vi "Import Export - Unflatten from XML (CAR fix).vi"(8 "Error In":errorcluster, 10 "XML String In":string) -> (0 "Error Out":errorcluster, 2 "Import":T1 {"Tree"."Properties"."Type" items=["K_STRING", "K_BOOL", "K_I32", "K_U32", "K_DOUBLE", "K_U64", "K_VARIANT", "K_DEPENDENTFILE", "K_DEPENDENTNODE", "K_DATASOURCENODE", "K_U16", "K_DBLARR", "K_U32ARR", "K_I32ARR", "K_STRINGARR", "K_DICTIONARY", "K_DICTIONARYARR"]})   [LabVIEW 2017, in "PXImc System Explorer.lvlib"]
doc: "Unflattern XML to Import data. It contains a workaround the CAR #198717."
uses:
  PXImc System Explorer.lvlib
  <vilib>/NI/NI VeriStand Advanced SysDef API/_Types/SysDef.Export.ctl
  <vilib>/NI/NI VeriStand Advanced SysDef API/_Types/TreeItem.ctl
  <vilib>/NI/NI VeriStand Advanced SysDef API/_Types/TreeItem.Info.ctl
  <vilib>/NI Veristand/Custom Device API/Custom Device Channel.ctl
  <vilib>/NI Veristand/Custom Device API/Custom Device Channel Type.ctl
  <vilib>/NI Veristand/Custom Device API/Custom Device Waveform.ctl
  <vilib>/NI Veristand/Custom Device API/Custom Device Waveform DataType.ctl
  <vilib>/NI/NI VeriStand Advanced SysDef API/_Types/TreeItem.Property.ctl
  <vilib>/NI VeriStand/Custom Device API/Custom Device API.lvlib
  <vilib>/NI/NI VeriStand Advanced SysDef API/SysDef API/Advanced System Definition.lvlib
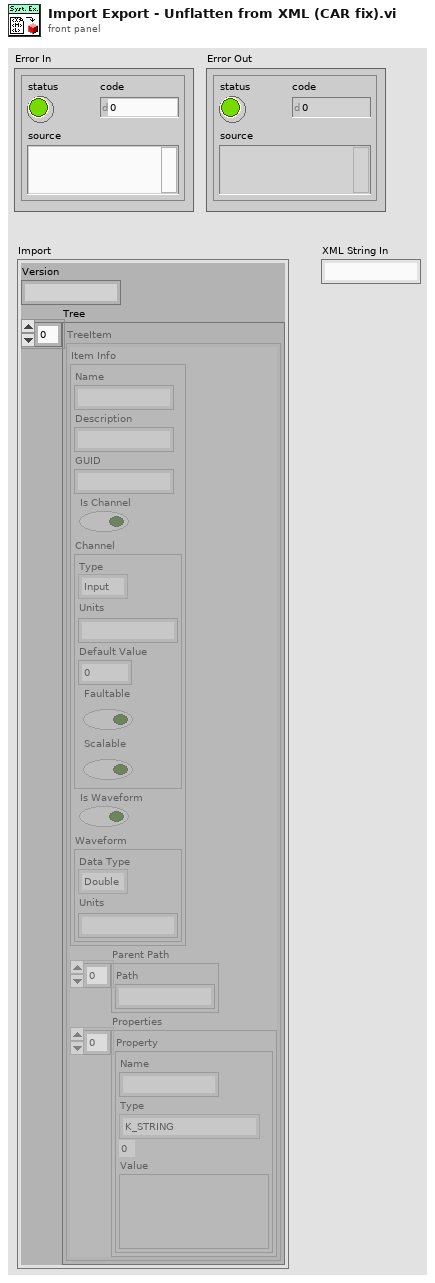
[diagram p1: front panel]
types:
  T1 = typedef "Advanced System Definition.lvlib/SysDef.Export.ctl" = cluster{"Version":string, "Tree":T2[]}
  T2 = typedef "Advanced System Definition.lvlib/TreeItem.ctl" = cluster{"Item Info":T3, "Parent Path":string[], "Properties":T8[]}
  T3 = typedef "Advanced System Definition.lvlib/TreeItem.Info.ctl" = cluster{"Name":string, "Description":string, "GUID":string, "Is Channel":bool, "Channel":T4, "Is Waveform":bool, "Waveform":T6}
  T4 = typedef "Custom Device API.lvlib/Custom Device Channel.ctl" = cluster{"Type":T5, "Units":string, "Default Value":dbl, "Faultable":bool, "Scalable":bool}
  T5 = typedef "Custom Device API.lvlib/Custom Device Channel Type.ctl" = enum16{"Input", "Output"}
  T6 = typedef "Custom Device API.lvlib/Custom Device Waveform.ctl" = cluster{"Data Type":T7, "Units":string}
  T7 = typedef "Custom Device API.lvlib/Custom Device Waveform DataType.ctl" = enum16{"Double", "Complex Double"}
  T8 = typedef "Advanced System Definition.lvlib/TreeItem.Property.ctl" = cluster{"Name":string, "Type":i32, "Value":variant}
  T9 = cluster{"Version":string, cluster{"Item Info":T3, "Parent Path":string[], cluster{"Name":string, "Type":i32, cluster{"type string":i16[], "data string":string}}[]}[]}
  T10 = cluster{"Item Info":T3, "Parent Path":string[], cluster{"Name":string, "Type":i32, cluster{"type string":i16[], "data string":string}}[]}[]
  T11 = cluster{"Name":string, "Type":i32, cluster{"type string":i16[], "data string":string}}[]
  T12 = cluster{"type string":i16[], "data string":string}
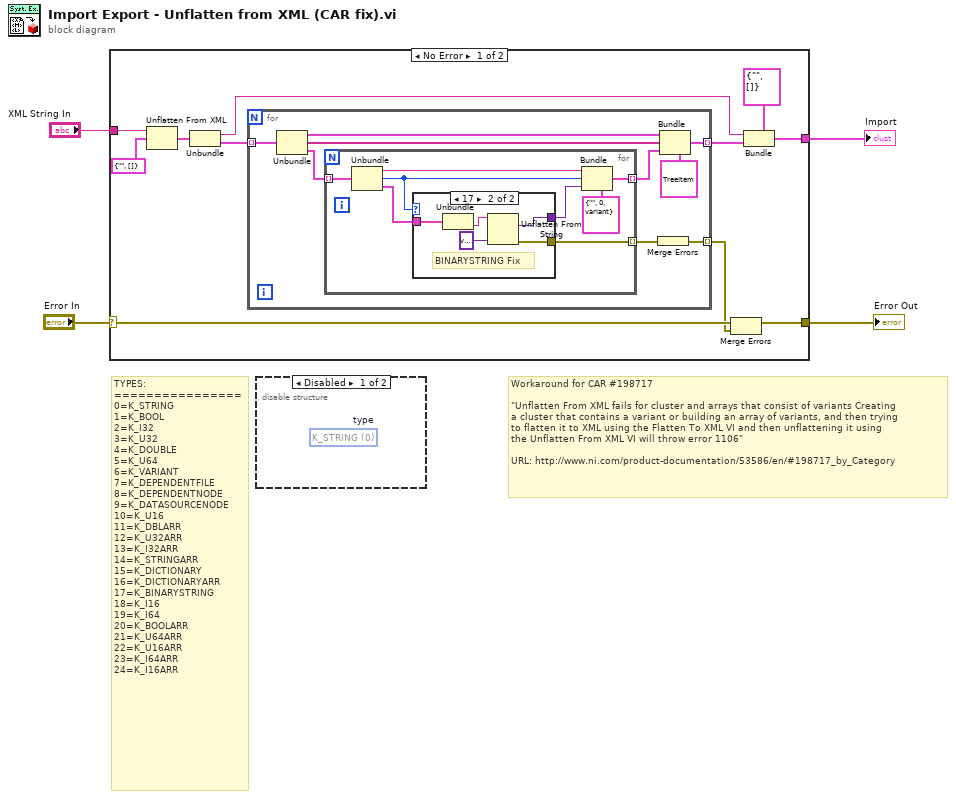
[diagram p0: block diagram]
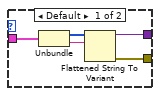
[diagram p2: hidden frame]
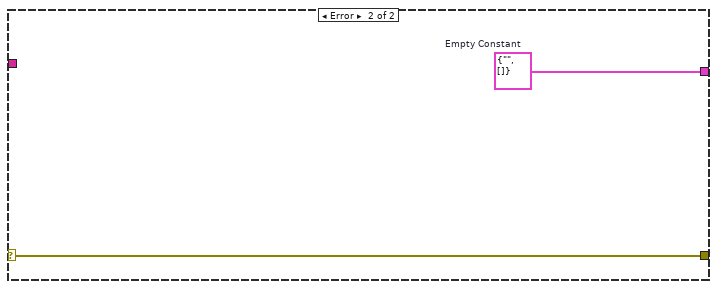
[diagram p3: hidden frame]
diagram:
  # "Workaround for CAR #198717\n\n\"Unflatten From XML fails for cluster and arrays that consist of variants Creating\na cluster that contains a variant or building an array of variants, and then trying\nto flatten it to XML using the Flatten To XML VI and then unflattening it using\nthe Unflatten From XML VI will throw error 1106\"\n\nURL: http://www.ni.com/product-documentation/53586/en/#198717_by_Category"
  # "TYPES:\n================\n0=K_STRING\n1=K_BOOL\n2=K_I32\n3=K_U32\n4=K_DOUBLE\n5=K_U64\n6=K_VARIANT\n7=K_DEPENDENTFILE\n8=K_DEPENDENTNODE\n9=K_DATASOURCENODE\n10=K_U16\n11=K_DBLARR\n12=K_U32ARR\n13=K_I32ARR\n14=K_STRINGARR\n15=K_DICTIONARY\n16=K_DICTIONARYARR\n17=K_BINARYSTRING\n18=K_I16\n19=K_I64\n20=K_BOOLARR\n21=K_U64ARR\n22=K_U16ARR\n23=K_I64ARR\n24=K_I16ARR"
  n1 = case shown="No Error" "Error In" {
    selector: "Error In" -> [w9 w44]
    tunnel: [w8 w44] -> w3
    tunnel: "XML String In" -> [w12 _]
    tunnel: [w6 w43] -> w1
    frame No Error {
      n2 = Unflatten From XML(xml string=w12, type=T9 {"Version"="", []} ("cluster")) -> (value=w11:T9)  [unwired: 1 in, 1 out]
      n3 = Unbundle(w11) -> ("Version"=w13:string, w15:T10)
      n4 = for {
        tunnel: w15 -> [w24] mode=indexing
        tunnel: [w21] -> w14 mode=indexing
        tunnel: [w16] -> w7 mode=indexing
        n5 = Unbundle(w24) -> ("Item Info"=w23:T3, "Parent Path"=w22:string[], w20:T11)
        n6 = for {
          tunnel: w20 -> [w32] mode=indexing
          tunnel: [w31] -> w19 mode=indexing
          tunnel: [w26] -> w17 mode=indexing
          n7 = Unbundle(w32) -> ("Name"=w30:string, "Type"=w25:i32, w28:T12)
          n8 = case shown="17" w25 {
            tunnel: w28 -> [w37 w42]
            tunnel: [w35 w38] -> w27
            tunnel: [w34 w41] -> w26
            frame Default {
              n9 = Unbundle(w37) -> ("type string"=w33:i16[], "data string"=w36:string)
              n10 = Flattened String To Variant(6:w36, 7:w33) -> (0:w34:errorcluster, 3:w35:variant)  [unwired: 1 in]
            }
            frame 17 {
              # "BINARYSTRING Fix"
              n11 = Unbundle(w42) -> ("data string"=w40:string)  [unwired: 1 out]
              n12 = Unflatten From String(type=variant ("Variant"), binary string=w40) -> (value=w38:variant, error out=w41:errorcluster)  [unwired: 3 in, 1 out]
            }
          }
          n13 = Bundle(cluster=T8 {"Name"="", "Type"=0, "Value"=variant(string "")} ("Property"), "Name"=w30, "Type"=w25, "Value"=w27) -> (w31:T8)
        }
        n14 = Merge Errors(w17) -> (w16:errorcluster)
        n15 = Bundle(cluster=T2 {"Item Info"={"Name"="", "Description"="", "GUID"="", "Is Channel"=FALSE, "Channel"={"Type"=enum."Input", "Units"="", "Default Value"=0.0, "Faultable"=FALSE, "Scalable"=FALSE}, "Is Waveform"=FALSE, "Waveform"={"Data Type"=enum."Double", "Units"=""}}, "Parent Path"=[], "Properties"=[]} ("TreeItem"), "Item Info"=w23, "Parent Path"=w22, "Properties"=w19) -> (w21:T2)
      }
      n16 = Merge Errors(w9, w7) -> (w8:errorcluster)
      n17 = Bundle(cluster=T1 {"Version"="", "Tree"=[]} ("Export"), "Version"=w13, "Tree"=w14) -> (w6:T1)
    }
    frame Error {
      w43 = T1 {"Version"="", "Tree"=[]}  # Empty Constant
    }
  }
  "Import" <- w1
  "Error Out" <- w3
  n18 = disable-structure shown="Disabled" {
    frame Disabled {
      (unwired) 0 items=["K_STRING", "K_BOOL", "K_I32", "K_U32", "K_DOUBLE", "K_U64", "K_VARIANT", "K_DEPENDENTFILE", "K_DEPENDENTNODE", "K_DATASOURCENODE", "K_U16", "K_DBLARR", "K_U32ARR", "K_I32ARR", "K_STRINGARR", "K_DICTIONARY", "K_DICTIONARYARR", "K_BINARYSTRING", "K_I16", "K_I64", "K_BOOLARR", "K_U64ARR", "K_U16ARR", "K_I64ARR", "K_I16ARR"]  # type
    }
    frame Enabled {
    }
  }
